vi "SDO_TRAJ_CALC_ORIENTATION.vi"(5 "Starting Fraction":dbl=0.25, 6 "Init":bool, 7 "Completion Fraction":dbl=0.75, 8 "Total Trajectory Time Sec":dbl, 9 "Elapsed Traj Time Sec":dbl, 10 "End Orientation Demand DEG":dbl, 11 "Starting Orientation  DEG":dbl) -> (1 "Rotational Velocity Rad Per Sec":dbl, 2 "Orientation Demand Deg":dbl, 3 "Orientation Demand":T1 {"SIN" format="%13.4f"; "COS" format="%13.4f"; "VALUE" format="%13.4f"})   [LabVIEW 2019]
uses:
  <vilib>/Rock Robotics/WPI/ThirdParty/JAS_Junk/TrajLib/TypeDef/ROTATION2D.ctl
  <vilib>/Rock Robotics/WPI/ThirdParty/JAS_Junk/TrajLib/Conv_Deg_Radians.vi
  <vilib>/Rock Robotics/WPI/ThirdParty/JAS_Junk/TrajLib/Rotation2d_CreateAngle.vi
  <vilib>/Rock Robotics/WPI/ThirdParty/JAS_Junk/TrajLib/Rotation2d_Plus.vi
  <vilib>/Rock Robotics/WPI/ThirdParty/JAS_Junk/TrajLib/Rotation2d_Minus.vi
  <vilib>/Rock Robotics/WPI/ThirdParty/JAS_Junk/TrajLib/Rotation2d_Times.vi
  <vilib>/Rock Robotics/WPI/ThirdParty/JAS_Junk/TrajLib/Conv_Radians_Deg.vi
  <vilib>/Rock Robotics/WPI/ThirdParty/JAS_Junk/TrajLib/Rotation2d_RotateBy.vi
  <vilib>/Rock Robotics/WPI/ThirdParty/JAS_Junk/TrajLib/Rotation2d_UnaryMinus.vi
  <vilib>/Rock Robotics/WPI/ThirdParty/JAS_Junk/TrajLib/Rotation2d_CreateXY.vi
  <vilib>/Rock Robotics/WPI/ThirdParty/JAS_Junk/TrajLib/Util_CalcDist.vi
  <vilib>/Rock Robotics/WPI/ThirdParty/JAS_Junk/TrajLib/Trajectory_Library.lvlib
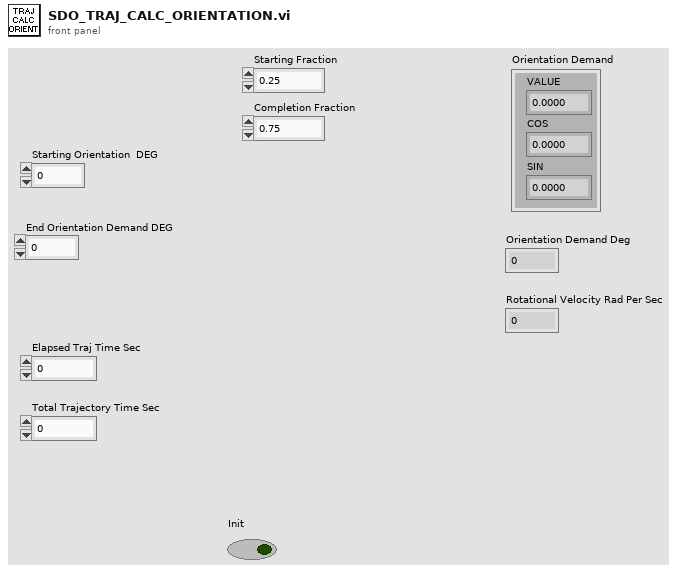
[diagram p1: front panel]
types:
  T1 = typedef "Trajectory_Library.lvlib/ROTATION2D.ctl" = cluster{"VALUE":dbl, "COS":dbl, "SIN":dbl}
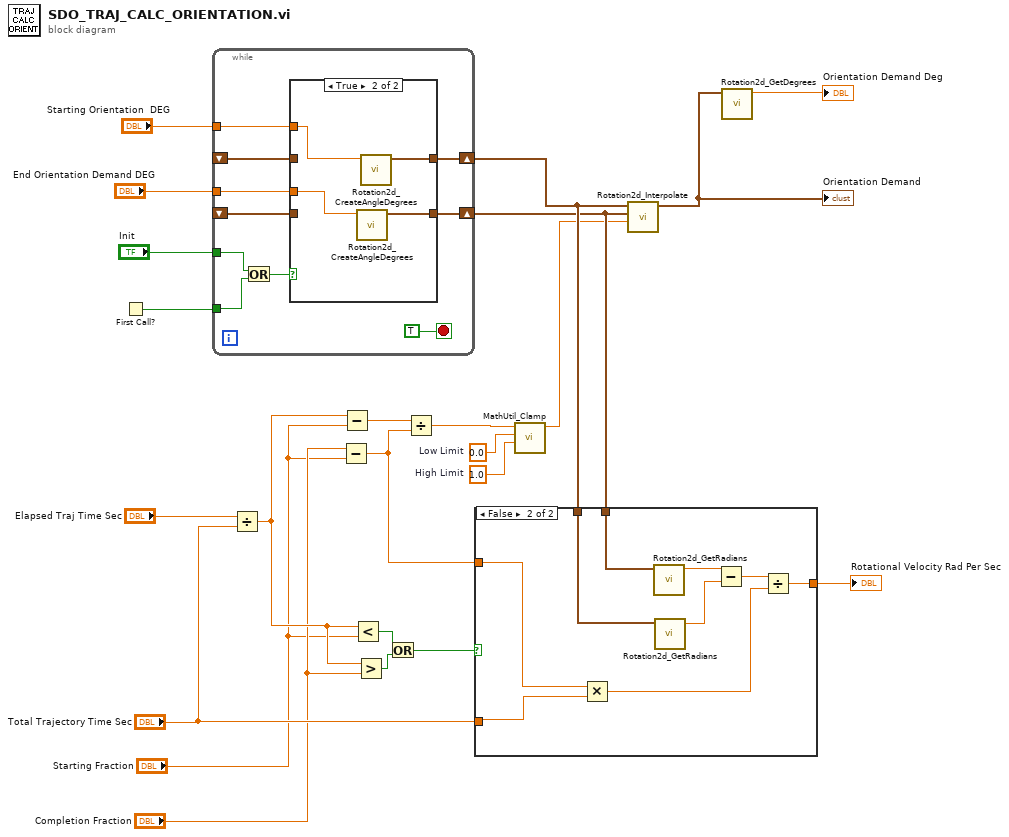
[diagram p0: block diagram]
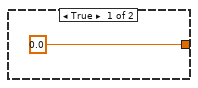
[diagram p2: hidden frame]
diagram:
  w6 = 1.0  # High Limit
  w5 = 0.0  # Low Limit
  n1 = First Call?() -> (First Call?: T/F=w1:bool)
  n2 = while {
    tunnel: "Init" -> [w25]
    tunnel: "End Orientation Demand DEG" -> [w32]
    shift-right: [w30] -> w16
    shift-left: _ -> [w28]
    shift-right: [w31] -> w17
    shift-left: _ -> [w29]
    tunnel: "Starting Orientation  DEG" -> [w27]
    tunnel: w1 -> [w24]
    stop <- TRUE stop-if-true
    n3 = Or(x=w25, y=w24) -> (x .or. y?=w26:bool)
    n4 = case shown="True" w26 {
      tunnel: w32 -> [_ w39]
      tunnel: [w35 w36] -> w31
      tunnel: [w34 w38] -> w30
      tunnel: w29 -> [w35 _]
      tunnel: w28 -> [w34 _]
      tunnel: w27 -> [_ w37]
      frame False {
      }
      frame True {
        n5 = call <vilib>:"Rotation2d_CreateAngleDegrees.vi"("Angle_Degrees"=w39) -> ("ROTATION"=w38:T1)  [unwired: 10 in]
        n6 = call <vilib>:"Rotation2d_CreateAngleDegrees.vi"("Angle_Degrees"=w37) -> ("ROTATION"=w36:T1)  [unwired: 10 in]
      }
    }
  }
  n7 = Divide(x="Elapsed Traj Time Sec", y="Total Trajectory Time Sec") -> (x/y=w9:dbl)
  n8 = Subtract(x="Completion Fraction", y="Starting Fraction") -> (x-y=w2:dbl)
  n9 = Subtract(x=w9, y="Starting Fraction") -> (x-y=w10:dbl)
  n10 = Less?(x=w9, y="Starting Fraction") -> (x < y?=w12:bool)
  n11 = Greater?(x=w9, y="Completion Fraction") -> (0:w13:bool)
  n12 = Or(x=w12, y=w13) -> (x .or. y?=w11:bool)
  n13 = Divide(x=w10, y=w2) -> (x/y=w4:dbl)
  n14 = case shown="False" w11 {
    tunnel: [0.0 w41] -> w19
    tunnel: w17 -> [_ w48]
    tunnel: w16 -> [_ w49]
    tunnel: "Total Trajectory Time Sec" -> [_ w43]
    tunnel: w2 -> [_ w44]
    frame True {
    }
    frame False {
      n15 = Multiply(x=w44, y=w43) -> (x*y=w42:dbl)
      n16 = call <vilib>:"Rotation2d_GetRadians.vi"("in ROTATION"=w49) -> ("AngleRadians"=w47:dbl)  [unwired: 10 in]
      n17 = call <vilib>:"Rotation2d_GetRadians.vi"("in ROTATION"=w48) -> ("AngleRadians"=w46:dbl)  [unwired: 10 in]
      n18 = Subtract(x=w47, y=w46) -> (x-y=w45:dbl)
      n19 = Divide(x=w45, y=w42) -> (x/y=w41:dbl)
    }
  }
  "Rotational Velocity Rad Per Sec" <- w19
  n20 = call <vilib>:"MathUtil_Clamp.vi"("High Limit"=w6, "Low Limit"=w5, "Value"=w4) -> ("Result"=w3:dbl)  [unwired: 8 in]
  n21 = call <vilib>:"Rotation2d_Interpolate.vi"("T"=w3, "EncValue ROTATION"=w16, "in ROTATION"=w17) -> ("Interpolated ROTATION"=w20:T1)  [unwired: 8 in]
  "Orientation Demand" <- w20
  n22 = call <vilib>:"Rotation2d_GetDegrees.vi"("in ROTATION"=w20) -> ("AngleDegrees"=→"Orientation Demand Deg":dbl)  [unwired: 10 in]
